vi "Add Pause Symbols to Tree.vi"(8 "error in":errorcluster, 11 "Data Tree Ref":refnum<vi>) -> (0 "error out":errorcluster)   [LabVIEW 2013, in "LVTM.lvlib"]
uses:
  LVTM.lvlib
  <vilib>/picture/picture.llb/imagedata.ctl
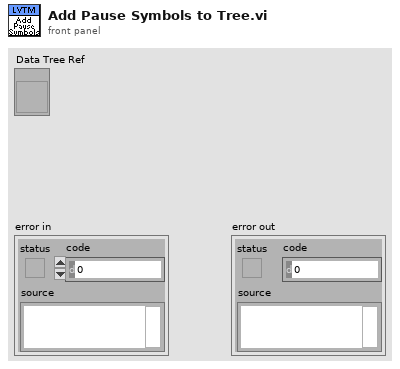
[diagram p1: front panel]
types:
  T1 = typedef "imagedata.ctl" = cluster{"image type":i32, "image depth":i32, "image":u8[], "mask":u8[], "colors":u32[], "Rectangle":cluster{"left":i16, "top":i16, "right":i16, "bottom":i16}}
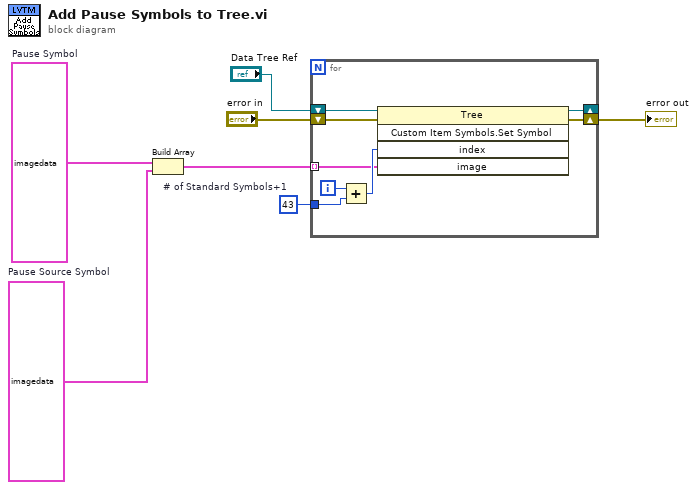
[diagram p0: block diagram]
diagram:
  w1 = T1 {"image type"=0, "image depth"=24, "image"=[28, 81, 128, 28, 81, 128, 28, 81, 128, 28, 81, 128, 28, 81, 128, 28, 81, 128, 28, 81, 128, 28, 81, 128, 28, 81, 128, 28, 81, 128, 28, 81, 128, 28, 81, 128, 28, 81, 128, 28, 81, 128, 237, 28, 36, 237, 28, 36, 237, 28, 36, 237, 28, 36, 237, 28, 36, 237, 28, 36, 237, 28, 36, 237, 28, 36, 237, 28, 36, 237, 28, 36, 237, 28, 36, 28, 81, 128, 28, 81, 128, 237, 28, 36, 51, 51, 51, 51, 51, 51, 51, 51, 51, 237, 28, 36, 237, 28, 36, 237, 28, 36, 51, 51, 51, 51, 51, 51, 51, 51, 51, 237, 28, 36, 28, 81, 128, 28, 81, 128, 237, 28, 36, 51, 51, 51, 51, 51, 51, 51, 51, 51, 237, 28, 36, 237, 28, 36, 237, 28, 36, 51, 51, 51, 51, 51, 51, 51, 51, 51, 237, 28, 36, 28, 81, 128, 28, 81, 128, 237, 28, 36, 51, 51, 51, 51, 51, 51, 51, 51, 51, 237, 28, 36, 237, 28, 36, 237, 28, 36, 51, 51, 51, 51, 51, 51, 51, 51, 51, 237, 28, 36, 28, 81, 128, 28, 81, 128, 237, 28, 36, 51, 51, 51, 51, 51, 51, 51, 51, 51, 237, 28, 36, 237, 28, 36, 237, 28, 36, 51, 51, 51, 51, 51, 51, 51, 51, 51, 237, 28, 36, 28, 81, 128, 28, 81, 128, 237, 28, 36, 51, 51, 51, 51, 51, 51, 51, 51, 51, 237, 28, 36, 237, 28, 36, 237, 28, 36, 51, 51, 51, 51, 51, 51, 51, 51, 51, 237, 28, 36, 28, 81, 128, 28, 81, 128, 237, 28, 36, 51, 51, 51, 51, 51, 51, 51, 51, 51, 237, 28, 36, 237, 28, 36, 237, 28, 36, 51, 51, 51, 51, 51, 51, 51, 51, 51, 237, 28, 36, 28, 81, 128, 28, 81, 128, 237, 28, 36, 51, 51, 51, 51, 51, 51, 51, 51, 51, 237, 28, 36, 237, 28, 36, 237, 28, 36, 51, 51, 51, 51, 51, 51, 51, 51, 51, 237, 28, 36, 28, 81, 128, 28, 81, 128, 237, 28, 36, 51, 51, 51, 51, 51, 51, 51, 51, 51, 237, 28, 36, 237, 28, 36, 237, 28, 36, 51, 51, 51, 51, 51, 51, 51, 51, 51, 237, 28, 36, 28, 81, 128, 28, 81, 128, 237, 28, 36, 51, 51, 51, 51, 51, 51, 51, 51, 51, 237, 28, 36, 237, 28, 36, 237, 28, 36, 51, 51, 51, 51, 51, 51, 51, 51, 51, 237, 28, 36, 28, 81, 128, 28, 81, 128, 237, 28, 36, 237, 28, 36, 237, 28, 36, 237, 28, 36, 237, 28, 36, 237, 28, 36, 237, 28, 36, 237, 28, 36, 237, 28, 36, 237, 28, 36, 237, 28, 36, 28, 81, 128, 28, 81, 128, 28, 81, 128, 28, 81, 128, 28, 81, 128, 28, 81, 128, 28, 81, 128, 28, 81, 128, 28, 81, 128, 28, 81, 128, 28, 81, 128, 28, 81, 128, 28, 81, 128, 28, 81, 128], "mask"=[], "colors"=[], "Rectangle"={"left"=0, "top"=0, "right"=13, "bottom"=13}}  # Pause Source Symbol
  w2 = T1 {"image type"=0, "image depth"=24, "image"=[28, 81, 128, 28, 81, 128, 28, 81, 128, 28, 81, 128, 28, 81, 128, 28, 81, 128, 28, 81, 128, 28, 81, 128, 28, 81, 128, 28, 81, 128, 28, 81, 128, 28, 81, 128, 28, 81, 128, 28, 81, 128, 255, 255, 255, 255, 255, 255, 255, 255, 255, 255, 255, 255, 255, 255, 255, 255, 255, 255, 255, 255, 255, 255, 255, 255, 255, 255, 255, 255, 255, 255, 255, 255, 255, 28, 81, 128, 28, 81, 128, 255, 255, 255, 51, 51, 51, 51, 51, 51, 51, 51, 51, 255, 255, 255, 255, 255, 255, 255, 255, 255, 51, 51, 51, 51, 51, 51, 51, 51, 51, 255, 255, 255, 28, 81, 128, 28, 81, 128, 255, 255, 255, 51, 51, 51, 51, 51, 51, 51, 51, 51, 255, 255, 255, 255, 255, 255, 255, 255, 255, 51, 51, 51, 51, 51, 51, 51, 51, 51, 255, 255, 255, 28, 81, 128, 28, 81, 128, 255, 255, 255, 51, 51, 51, 51, 51, 51, 51, 51, 51, 255, 255, 255, 255, 255, 255, 255, 255, 255, 51, 51, 51, 51, 51, 51, 51, 51, 51, 255, 255, 255, 28, 81, 128, 28, 81, 128, 255, 255, 255, 51, 51, 51, 51, 51, 51, 51, 51, 51, 255, 255, 255, 255, 255, 255, 255, 255, 255, 51, 51, 51, 51, 51, 51, 51, 51, 51, 255, 255, 255, 28, 81, 128, 28, 81, 128, 255, 255, 255, 51, 51, 51, 51, 51, 51, 51, 51, 51, 255, 255, 255, 255, 255, 255, 255, 255, 255, 51, 51, 51, 51, 51, 51, 51, 51, 51, 255, 255, 255, 28, 81, 128, 28, 81, 128, 255, 255, 255, 51, 51, 51, 51, 51, 51, 51, 51, 51, 255, 255, 255, 255, 255, 255, 255, 255, 255, 51, 51, 51, 51, 51, 51, 51, 51, 51, 255, 255, 255, 28, 81, 128, 28, 81, 128, 255, 255, 255, 51, 51, 51, 51, 51, 51, 51, 51, 51, 255, 255, 255, 255, 255, 255, 255, 255, 255, 51, 51, 51, 51, 51, 51, 51, 51, 51, 255, 255, 255, 28, 81, 128, 28, 81, 128, 255, 255, 255, 51, 51, 51, 51, 51, 51, 51, 51, 51, 255, 255, 255, 255, 255, 255, 255, 255, 255, 51, 51, 51, 51, 51, 51, 51, 51, 51, 255, 255, 255, 28, 81, 128, 28, 81, 128, 255, 255, 255, 51, 51, 51, 51, 51, 51, 51, 51, 51, 255, 255, 255, 255, 255, 255, 255, 255, 255, 51, 51, 51, 51, 51, 51, 51, 51, 51, 255, 255, 255, 28, 81, 128, 28, 81, 128, 255, 255, 255, 255, 255, 255, 255, 255, 255, 255, 255, 255, 255, 255, 255, 255, 255, 255, 255, 255, 255, 255, 255, 255, 255, 255, 255, 255, 255, 255, 255, 255, 255, 28, 81, 128, 28, 81, 128, 28, 81, 128, 28, 81, 128, 28, 81, 128, 28, 81, 128, 28, 81, 128, 28, 81, 128, 28, 81, 128, 28, 81, 128, 28, 81, 128, 28, 81, 128, 28, 81, 128, 28, 81, 128], "mask"=[], "colors"=[], "Rectangle"={"left"=0, "top"=0, "right"=13, "bottom"=13}}  # Pause Symbol
  w7 = 43  # # of Standard Symbols+1
  n1 = Build Array(w2, w1) -> (w3:T1[])
  n2 = for {
    tunnel: w7 -> [w14]
    shift-right: [w11] -> _
    shift-left: "Data Tree Ref" -> [w13]
    tunnel: w3 -> [w10] mode=indexing
    shift-right: [w8] -> w5
    shift-left: "error in" -> [w9]
    i -> [w15]
    n3 = Add(x=w15, y=w14) -> (x+y=w12:i32)
    n4 = invoke on="Invoke Node" class="Tree" method="Custom Item Symbols.Set Symbol"(reference=w13, error in=w9, "index"=w12, "image"=w10) -> (reference out=w11:refnum<vi>, error out=w8:errorcluster)  [unwired: 1 in, 3 out]
  }
  "error out" <- w5
